vi "Resistance_test_3.vi"() -> ()   [LabVIEW 2017]
uses:
  <vilib>/Utility/error.llb/DialogType.ctl
  <vilib>/DAQmx/read.llb/DAQmx Read (Analog 2D DBL NChan NSamp).vi
  <vilib>/DAQmx/read.llb/DAQmx Read (Analog 1D Wfm NChan NSamp).vi
  <vilib>/DAQmx/write.llb/DAQmx Write (Analog DBL 1Chan 1Samp).vi
  <vilib>/DAQmx/create/channels.llb/DAQmx Create Channel (AO-Voltage-Basic).vi
  <vilib>/DAQmx/create/channels.llb/DAQmx Create Channel (AI-Voltage-Basic).vi
  <vilib>/DAQmx/configure/timing.llb/DAQmx Timing (Sample Clock).vi
  <vilib>/DAQmx/configure/trigger.llb/DAQmx Start Trigger (None).vi
  <vilib>/DAQmx/miscellaneous.llb/DAQmx Fill In Error Info.vi
  <resource>/objmgr/daqmx.rc
panel:
  in  "Rsh":dbl=98.2 format="%0.1f"
  out "Average":dbl=2.454455125699035
  in  "samples per channel":i32=200000
  in  "rate":dbl=100000.0 format="%0.0f"
  out "MSE":dbl=0.004435206606928749
  out "size of buffer":i32=9984
  out "size(s)":i32=100
  in  "Number of points":i32=100
  out "Ush.Min":dbl=-0.5
  out "Ush.Max":dbl=0.5
  out "U.Min":dbl=-0.1
  out "U.Max":dbl=0.1
  in  "Voltage Output, V":dbl=0.5
  in  "ms to wait":u32=100
  out "AO.Max":dbl=0.5
  out "AO.Min":dbl
  in  "Error (in)":errorcluster
  in  "stop":bool
  out "SpectrumGraph":cluster{i32[], dbl[]}(graph)={[1, 2, 3, 4, 5, 6, 7, 8, 9, 10, 11, 12, 13, 14, 15, 16, 17, 18, 19, 20, 21, 22, 23, 24, 25, 26, 27, 28, 29, 30, 31, 32, 33, 34, 35, 36, 37, 38, 39, 40, 41, 42, 43, 44, 45, 46, 47, 48, 49, 50, 51, 52, 53, 54, 55, 56, 57, 58, 59, 60, 61, 62, 63, 64, 65, 66, 67, 68, 69, 70, 71, 72, 73, 74, 75, 76, 77, 78, 79, 80, 81, 82, 83, 84, 85, 86, 87, 88, 89, 90, 91, 92, 93, 94, 95, 96, 97, 98, 99, 100], [2.460272177612693, 2.4561198276109315, 2.452504654179395, 2.452578542575543, 2.4524286960414954, 2.4581957262597123, 2.4500878968066147, 2.4612772241882217, 2.448195548138903, 2.451971478505558, 2.450932398639929, 2.444450709731608, 2.4515795757065613, 2.4566874887186, 2.4511589813413397, 2.453476777607862, 2.457816358046222, 2.452959719180252, 2.45674279457507, 2.4536051593157366, 2.4476150112190056, 2.447481739942543, 2.4555534689913707, 2.457497178810143, 2.455003292024694, 2.4466757490513693, 2.4579083237186397, 2.4500218646842074, 2.453685143142287, 2.4512167599890904, 2.4545430731181495, 2.4543480780463645, 2.451766409982298, 2.4570629564421074, 2.450206780187229, 2.4547758121087218, 2.4591520163246465, 2.46282811928863, 2.4492398539214326, 2.4530738523987545, 2.4467585147196074, 2.4569469576280976, 2.4631804138318127, 2.461644960285589, 2.4519676177499936, 2.4564617821339767, 2.452378700872091, 2.4598234637782435, 2.458661023349093, 2.459016197728431, 2.4545299810350887, 2.4553451158381185, 2.457301188443594, 2.4486629031453893, 2.456376058144437, 2.4566047278157215, 2.4523204222875554, 2.453813271339721, 2.451675467434209, 2.448109263066983, 2.4613890637885305, 2.451902116478789, 2.4551344777967437, 2.465328778984662, 2.454809892466976, 2.4543581062482267, 2.4523119577383183, 2.458768572481827, 2.458910451800771, 2.4524533976776195, 2.461112812830327, 2.4459630495645808, 2.444418948719615, 2.4563478984624, 2.4589407401168746, 2.4575536597208854, 2.4497444426986883, 2.4555646853582234, 2.454784666241629, 2.44572494935055, 2.4598990299959933, 2.4618857220388017, 2.449895942822891, 2.4574198445735616, 2.4509636900612604, 2.451871354101766, 2.4486366973122355, 2.452260832265065, 2.4553560282742475, 2.4614177730815365, 2.4573246656143315, 2.4510933987984913, 2.4589888353948215, 2.452509004295127, 2.456672563705906, 2.4544962583854932, 2.4592027334878415, 2.4540407628994254, 2.452160971733344, 2.4596185437334377]}
  out "error out":errorcluster
  in  "DAQ channel In Voltage Output":tag="DAQ6363/ao0"
  in  "DAQ channel In Voltage U":tag="DAQ6363/ai5"
  in  "DAQ channel In Voltage Ush":tag="DAQ6363/ai4"
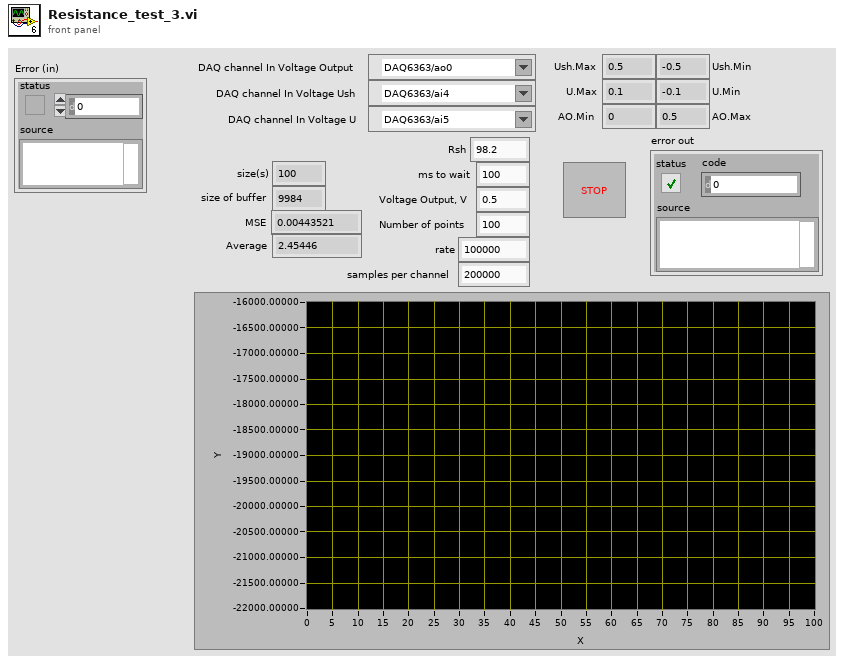
[diagram p1: front panel]
types:
  T1 = typedef "DialogType.ctl" = u16
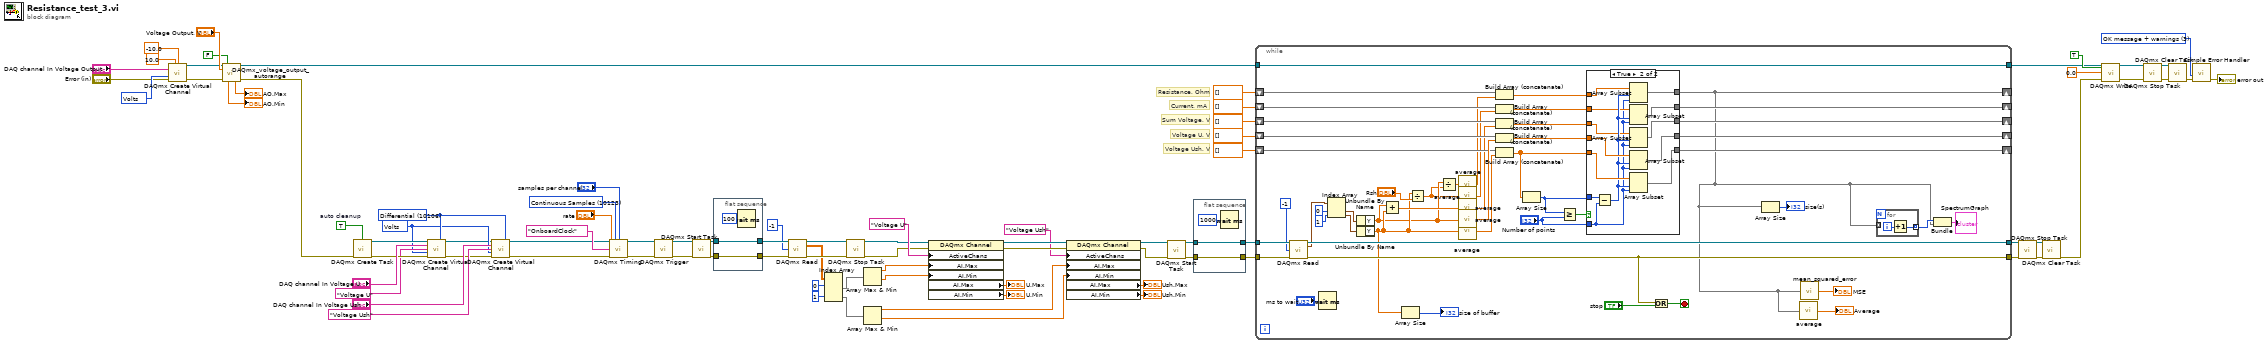
[diagram p0: block diagram]
diagram:
  w51 = 10348 items=["Volts"=10348, "From Custom Scale"=10065] ("units")
  w77 = TRUE  # auto cleanup
  w81 = T1 3 items=["no dialog", "OK message", "continue or stop message", "OK message + warnings", "continue/stop + warnings"] ("type of dialog (OK msg:1)")
  w85 = 10123 items=["Finite Samples"=10178, "Continuous Samples"=10123, "Hardware Timed Single Point"=12522] ("sample mode")
  w12 = 10106 items=["Default"=-1, "RSE"=10083, "NRSE"=10078, "Differential"=10106, "Pseudodifferential"=12529] ("input terminal configuration")
  w11 = 10348 items=["Volts"=10348, "From Custom Scale"=10065] ("units")
  # "Sum Voltage, V"
  # "Current, mA"
  # "Resistance, Ohm"
  # "Voltage Ush, V"
  # "Voltage U, V"
  n1 = call-poly <vilib>:"DAQmx Create Virtual Channel.vi"("maximum value"=10.0, "minimum value"=-10.0, "physical channels"="DAQ channel In Voltage Output", "units"=w51, "error in"="Error (in)") -> ("task out"=w55:refnum<k21>, "error out"=w56:errorcluster)  [unwired: 9 in]
  n2 = call "DAQmx_voltage_output_autorange.vi"("DAQ task Voltage Output in"=w55, "Bipolar"=FALSE, "Voltage Output, V"="Voltage Output, V", "error in (no error)"=w56) -> ("DAQ task Voltage Output out"=w49:refnum<k21>, "AO.Min"=→"AO.Min":dbl, "AO.Max"=→"AO.Max":dbl, "error out"=w45:errorcluster)  [unwired: 8 in]
  n3 = call <vilib>:"DAQmx Create Task.vi"("auto cleanup"=w77, "error in"=w45) -> ("task out"=w76:refnum<k21>, "error out"=w75:errorcluster)  [unwired: 12 in]
  n4 = call-poly <vilib>:"DAQmx Create Virtual Channel.vi"("task in"=w76, "input terminal configuration"=w12, "physical channels"="DAQ channel In Voltage U", "name to assign"="Voltage U", "units"=w11, "error in"=w75) -> ("task out"=w6:refnum<k21>, "error out"=w5:errorcluster)  [unwired: 8 in]
  n5 = call-poly <vilib>:"DAQmx Create Virtual Channel.vi"("task in"=w6, "input terminal configuration"=w12, "physical channels"="DAQ channel In Voltage Ush", "name to assign"="Voltage Ush", "units"=w11, "error in"=w5) -> ("task out"=w73:refnum<k21>, "error out"=w72:errorcluster)  [unwired: 8 in]
  n6 = call-poly <vilib>:"DAQmx Timing.vi"("task/channels in"=w73, "sample mode"=w85, "samples per channel"="samples per channel", "rate"="rate", "source"=tag "OnboardClock", "error in"=w72) -> ("task out"=w71:refnum<k21>, "error out"=w70:errorcluster)  [unwired: 8 in]
  n7 = call-poly <vilib>:"DAQmx Trigger.vi"("task/channels in"=w71, "error in"=w70) -> ("task out"=w24:refnum<k21>, "error out"=w23:errorcluster)  [unwired: 12 in]
  n8 = call <vilib>:"DAQmx Start Task.vi"("task/channels in"=w24, "error in"=w23) -> ("task out"=w33:refnum<k21>, "error out"=w31:errorcluster)  [unwired: 12 in]
  n9 = flat-sequence {
    tunnel: w31 -> [w89]
    tunnel: [w89] -> w32
    tunnel: w33 -> [w88]
    tunnel: [w88] -> w34
    frame #0 {
      n10 = Wait (ms)(milliseconds to wait=u32 100) -> ()  [unwired: 1 out]
    }
  }
  n11 = call-poly <vilib>:"DAQmx Read.vi"("task/channels in"=w34, "number of samples per channel"=-1, "error in"=w32) -> ("task out"=w28:refnum<k21>, "data"=w27:dbl[][], "error out"=w29:errorcluster)  [unwired: 10 in]
  n12 = Index Array(array=w27, index (row) #1=0 ("index"), index (row) #2=1 ("index")) -> (element #1=w35:dbl[], element #2=w36:dbl[])  [unwired: 2 in]
  n13 = call <vilib>:"DAQmx Stop Task.vi"("task/channels in"=w28, "error in"=w29) -> ("task out"=w22:refnum<k21>, "error out"=w21:errorcluster)  [unwired: 12 in]
  n14 = Array Max & Min(array=w35) -> (max value=w20:dbl, min value=w19:dbl)  [unwired: 2 out]
  n15 = Array Max & Min(array=w36) -> (max value=w10:dbl, min value=w9:dbl)  [unwired: 2 out]
  n16 = property class="DAQmx Channel"(reference=w22, error in=w21, "ActiveChans"="Voltage U", "AI.Max"=w20, "AI.Min"=w19) -> (reference out=w61:refnum<k21>, error out=w60:errorcluster, "AI.Max"=→"U.Max":dbl, "AI.Min"=→"U.Min":dbl)
  n17 = property class="DAQmx Channel"(reference=w61, error in=w60, "ActiveChans"="Voltage Ush", "AI.Max"=w10, "AI.Min"=w9) -> (reference out=w8:refnum<k21>, error out=w7:errorcluster, "AI.Max"=→"Ush.Max":dbl, "AI.Min"=→"Ush.Min":dbl)
  n18 = call <vilib>:"DAQmx Start Task.vi"("task/channels in"=w8, "error in"=w7) -> ("task out"=w16:refnum<k21>, "error out"=w15:errorcluster)  [unwired: 12 in]
  n19 = flat-sequence {
    tunnel: w15 -> [w92]
    tunnel: [w92] -> w17
    tunnel: w16 -> [w91]
    tunnel: [w91] -> w18
    frame #0 {
      n20 = Wait (ms)(milliseconds to wait=u32 1000) -> ()  [unwired: 1 out]
    }
  }
  n21 = while {
    tunnel: w18 -> [w141]
    tunnel: w17 -> [w139]
    tunnel: [w130] -> w69
    tunnel: [w138] -> w68
    tunnel: w49 -> [w131]
    tunnel: [w131] -> w48
    shift-right: [w95] -> _
    shift-left: dbl[] [] -> [w126]
    shift-right: [w94] -> _
    shift-left: dbl[] [] -> [w125]
    shift-right: [w93] -> _
    shift-left: dbl[] [] -> [w107]
    shift-right: [w97] -> _
    shift-left: dbl[] [] -> [w108]
    shift-right: [w96] -> _
    shift-left: dbl[] [] -> [w109]
    stop <- w128 stop-if-true
    n22 = call-poly <vilib>:"DAQmx Read.vi"("task/channels in"=w141, "number of samples per channel"=-1, "error in"=w139) -> ("task out"=w138:refnum<k21>, "data"=w137:waveform(dbl)[], "error out"=w130:errorcluster)  [unwired: 10 in]
    n23 = Wait (ms)(milliseconds to wait="ms to wait") -> ()  [unwired: 1 out]
    n24 = Index Array(array=w137, index #1=0 ("index"), index #2=1 ("index")) -> (element #1=w134:waveform(dbl), element #2=w133:waveform(dbl))
    n25 = Unbundle By Name(w134) -> ("Y"=w112:dbl[])
    n26 = Unbundle By Name(w133) -> ("Y"=w113:dbl[])
    n27 = Add(x=w112, y=w113) -> (x+y=w115:dbl[])
    n28 = Array Size(array=w113) -> (size(s)=→"size of buffer":i32)
    n29 = Divide(x=w113, y="Rsh") -> (x/y=w111:dbl[])
    n30 = Divide(x=w112, y=w111) -> (x/y=w110:dbl[])
    n31 = call "average.vi"("Array"=w110) -> ("Average"=w104:dbl)
    n32 = call "average.vi"("Array"=w111) -> ("Average"=w105:dbl)
    n33 = call "average.vi"("Array"=w115) -> ("Average"=w106:dbl)
    n34 = call "average.vi"("Array"=w112) -> ("Average"=w127:dbl)
    n35 = call "average.vi"("Array"=w113) -> ("Average"=w124:dbl)
    n36 = Build Array (concatenate)(w107, w104) -> (w101:dbl[])
    n37 = Build Array (concatenate)(w108, w105) -> (w102:dbl[])
    n38 = Build Array (concatenate)(w109, w106) -> (w103:dbl[])
    n39 = Build Array (concatenate)(w126, w127) -> (w123:dbl[])
    n40 = Build Array (concatenate)(w125, w124) -> (w100:dbl[])
    n41 = Array Size(array=w100) -> (size(s)=w121:i32)
    n42 = Greater Or Equal?(x=w121, y="Number of points") -> (x >= y?=w122:bool)
    n43 = case shown="True" w122 {
      tunnel: [w146 w159] -> w95
      tunnel: w123 -> [w146 w158]
      tunnel: w100 -> [w145 w156]
      tunnel: w121 -> [_ w157]
      tunnel: "Number of points" -> [_ w150]
      tunnel: [w145 w155] -> w94
      tunnel: w103 -> [w142 w151]
      tunnel: w102 -> [w143 w152]
      tunnel: w101 -> [w144 w153]
      tunnel: [w142 w149] -> w96
      tunnel: [w143 w148] -> w97
      tunnel: [w144 w147] -> w93
      frame False {
      }
      frame True {
        n44 = Subtract(x=w157, y=w150) -> (x-y=w154:i32)
        n45 = Array Subset(array=w153, index=w154, length=w150) -> (w147:dbl[])
        n46 = Array Subset(array=w152, index=w154, length=w150) -> (w148:dbl[])
        n47 = Array Subset(array=w151, index=w154, length=w150) -> (w149:dbl[])
        n48 = Array Subset(array=w158, index=w154, length=w150) -> (w159:dbl[])
        n49 = Array Subset(array=w156, index=w154, length=w150) -> (w155:dbl[])
      }
    }
    n50 = Or(x=w130, y="stop") -> (x .or. y?=w128:bool)
    n51 = Array Size(array=w93) -> (size(s)=→"size(s)":i32)
    n52 = call "average.vi"("Array"=w93) -> ("Average"=→"Average":dbl)
    n53 = call "mean_squared_error.vi"("Array"=w93) -> ("Mean Squared Error"=→"MSE":dbl)
    n54 = for {
      tunnel: [w160] -> w119 mode=indexing
      tunnel: w93 -> [_] mode=indexing
      i -> [w161]
      n55 = Increment(x=w161) -> (x+1=w160:i32)
    }
    n56 = Bundle(w119, w93) -> (→"SpectrumGraph":cluster{i32[], dbl[]})  [unwired: 1 in]
  }
  n57 = call <vilib>:"DAQmx Stop Task.vi"("task/channels in"=w68, "error in"=w69) -> ("task out"=w83:refnum<k21>, "error out"=w84:errorcluster)  [unwired: 12 in]
  n58 = call <vilib>:"DAQmx Clear Task.vi"("task in"=w83, "error in"=w84) -> ("error out"=w47:errorcluster)  [unwired: 13 in]
  n59 = call-poly <vilib>:"DAQmx Write.vi"("task/channels in"=w48, "auto start"=TRUE, "data"=0.0, "error in"=w47) -> ("task out"=w66:refnum<k21>, "error out"=w67:errorcluster)  [unwired: 9 in, 1 out]
  n60 = call <vilib>:"DAQmx Stop Task.vi"("task/channels in"=w66, "error in"=w67) -> ("task out"=w79:refnum<k21>, "error out"=w80:errorcluster)  [unwired: 12 in]
  n61 = call <vilib>:"DAQmx Clear Task.vi"("task in"=w79, "error in"=w80) -> ("error out"=w46:errorcluster)  [unwired: 13 in]
  n62 = call <vilib>:"Simple Error Handler.vi"("type of dialog (OK msg:1)"=w81, "error in (no error)"=w46) -> ("error out"=→"error out":errorcluster)  [unwired: 3 in, 4 out]
